vi "xml_test_2.vi"() -> ()   [LabVIEW 2010]
uses:
  <vilib>/Utility/xml.llb/Read From XML File(array).vi
  <vilib>/Utility/xml.llb/Write to XML File(string).vi
panel:
  out "Array":cluster{"String":string, "Numeric":dbl}[](array[cluster])
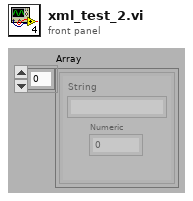
[diagram p1: front panel]
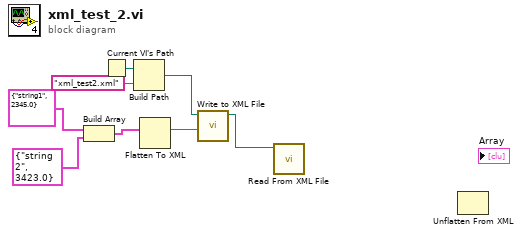
[diagram p0: block diagram]
diagram:
  n1 = Build Array(cluster{"String":string, "Numeric":dbl} {"String"="string1", "Numeric"=2345.0} ("Cluster"), cluster{"String":string, "Numeric":dbl} {"String"="string 2", "Numeric"=3423.0} ("Cluster")) -> (w6:cluster{"String":string, "Numeric":dbl}[])
  n2 = Current VI's Path() -> (path=w4:path)
  n3 = Build Path(base path=w4, name or relative path="xml_test2.xml") -> (appended path=w2:path)
  n4 = Flatten To XML(anything=w6) -> (xml string=w5:string)
  n5 = call-poly <vilib>:"Write to XML File.vi"("XML Input"=w5, "XML File Path"=w2) -> ("XML File Path(duplicate)"=w1:path)  [unwired: 7 in, 2 out]
  n6 = call-poly <vilib>:"Read From XML File.vi"("XML File Path"=w1) -> ()  [unwired: 8 in, 3 out]
  n7 = Unflatten From XML() -> ()  [unwired: 3 in, 2 out]
